vi "myRIO__TCP_readAccumParse_getCmd_1st.vi"(10 "input_count":i32, 11 "input_strAccum":string) -> (0 "output_countCmd":i32, 1 "output_strCmd":string, 2 "output_count":i32, 3 "output_strAccum":string, 4 "output_haveCmd":bool)   [LabVIEW 2014]
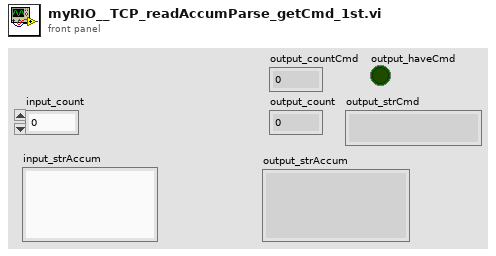
[diagram p1: front panel]
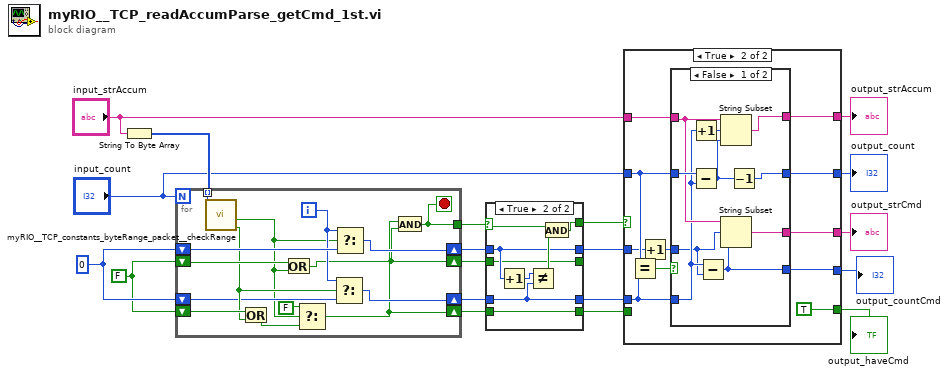
[diagram p0: block diagram]
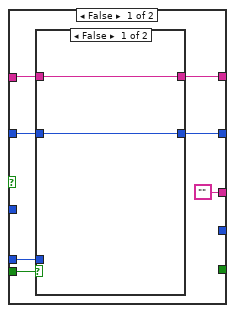
[diagram p2: hidden frame]
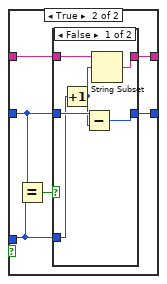
[diagram p3: hidden frame]
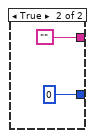
[diagram p4: hidden frame]
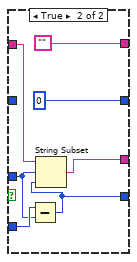
[diagram p5: hidden frame]
diagram:
  w17 = FALSE
  w18 = 0
  n1 = String To Byte Array(string="input_strAccum") -> (unsigned byte array=w19:u8[])
  n2 = for {
    N: "input_count" -> [_]
    tunnel: w19 -> [w34] mode=indexing
    shift-right: [w27] -> w15
    shift-left: w18 -> [w31]
    shift-right: [w26] -> w13
    shift-left: w18 -> [w29]
    shift-right: [w25] -> w14
    shift-left: w17 -> [w33]
    shift-right: [w20] -> w12
    shift-left: w17 -> [w32]
    tunnel: [w24] -> w16
    i -> [w28]
    stop <- w24 stop-if-true
    n3 = call "myRIO__TCP_constants_byteRange_packet__checkRange.vi"("input_byte"=w34) -> ("output_packet_end"=w30:bool, "output_packet_start"=w23:bool)  [unwired: 8 in, 1 out]
    n4 = Or(x=w32, y=w30) -> (x .or. y?=w21:bool)
    n5 = Or(x=w33, y=w23) -> (x .or. y?=w25:bool)
    n6 = Select(t=FALSE, s=w23, f=w21) -> (s? t:f=w20:bool)
    n7 = Select(t=w28, s=w30, f=w29) -> (s? t:f=w26:i32)
    n8 = Select(t=w28, s=w23, f=w31) -> (s? t:f=w27:i32)
    n9 = And(x=w20, y=w25) -> (x .and. y?=w24:bool)
  }
  n10 = case shown="True" w16 {
    selector: w16 -> [w35 w46]
    tunnel: w15 -> [w39 w43]
    tunnel: [w39 w43] -> w6
    tunnel: w14 -> [w38 w42]
    tunnel: [w38 w42] -> _
    tunnel: w13 -> [w37 w41]
    tunnel: [w37 w41] -> w9
    tunnel: w12 -> [w36 w40]
    tunnel: [w36 w40] -> w10
    tunnel: [w35 w44] -> w11
    frame False {
    }
    frame True {
      n11 = Increment(x=w43) -> (x+1=w47:i32)
      n12 = Not Equal?(x=w47, y=w41) -> (x != y?=w45:bool)
      n13 = And(x=w46, y=w45) -> (x .and. y?=w44:bool)
    }
  }
  n14 = case shown="True" w11 {
    tunnel: w10 -> [w54 _]
    tunnel: w9 -> [w53 w75]
    tunnel: "input_strAccum" -> [w51 w78]
    tunnel: "input_count" -> [w52 w74]
    tunnel: [w50 w79] -> w4
    tunnel: [w49 w80] -> w5
    tunnel: ["" w77] -> w3
    tunnel: w6 -> [_ w73]
    tunnel: [_ TRUE] -> w2
    tunnel: [_ w71] -> w1
    frame False {
      n15 = case shown="False" w54 {
        tunnel: w53 -> [_ w60]
        tunnel: w52 -> [w56 w59]
        tunnel: w51 -> [w55 w61]
        tunnel: [w56 w57] -> w50
        tunnel: [w55 w58] -> w49
        frame False {
        }
        frame True {
          n16 = Equal?(x=w59, y=w60) -> (x = y?=w62:bool)
          n17 = case shown="False" w62 {
            tunnel: w61 -> [w68 _]
            tunnel: w60 -> [w66 _]
            tunnel: w59 -> [w67 _]
            tunnel: [w64 ""] -> w58
            tunnel: [w65 0] -> w57
            frame False {
              n18 = Increment(x=w66) -> (x+1=w63:i32)
              n19 = Subtract(x=w67, y=w63) -> (x-y=w65:i32)
              n20 = String Subset(string=w68, offset (0)=w63) -> (substring=w64:string)  [unwired: 1 in]
            }
            frame True {
            }
          }
        }
      }
    }
    frame True {
      n21 = Equal?(x=w74, y=w75) -> (x = y?=w81:bool)
      n22 = Increment(x=w73) -> (x+1=w72:i32)
      n23 = case shown="False" w81 {
        tunnel: [w89 ""] -> w80
        tunnel: [w82 0] -> w79
        tunnel: w78 -> [w88 w96]
        tunnel: w72 -> [w85 w93]
        tunnel: [w87 w95] -> w77
        tunnel: w75 -> [w86 w94]
        tunnel: w74 -> [w90 _]
        tunnel: [w84 w92] -> w71
        frame False {
          n24 = Increment(x=w86) -> (x+1=w91:i32)
          n25 = Subtract(x=w90, y=w86) -> (x-y=w83:i32)
          n26 = Subtract(x=w86, y=w85) -> (x-y=w84:i32)
          n27 = String Subset(string=w88, offset (0)=w91, length (rest)=w83) -> (substring=w89:string)
          n28 = String Subset(string=w88, offset (0)=w85, length (rest)=w84) -> (substring=w87:string)
          n29 = Decrement(x=w83) -> (x-1=w82:i32)
        }
        frame True {
          n30 = Subtract(x=w94, y=w93) -> (x-y=w92:i32)
          n31 = String Subset(string=w96, offset (0)=w93, length (rest)=w92) -> (substring=w95:string)
        }
      }
    }
  }
  "output_strAccum" <- w5
  "output_count" <- w4
  "output_strCmd" <- w3
  "output_haveCmd" <- w2
  "output_countCmd" <- w1
